vi "Excersie_3.vi"() -> ()   [LabVIEW 2013]
panel:
  in  "Slide":dbl(slide) scale=0.0..2000.0
  in  "stop":bool
  out "Waveform Chart":dbl(graph)
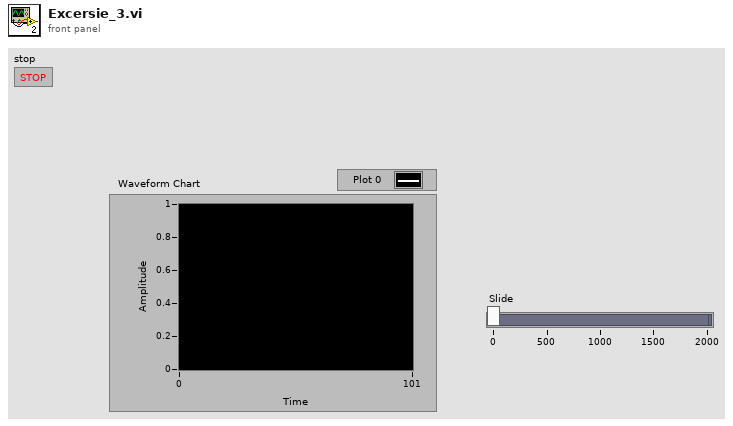
[diagram p1: front panel]
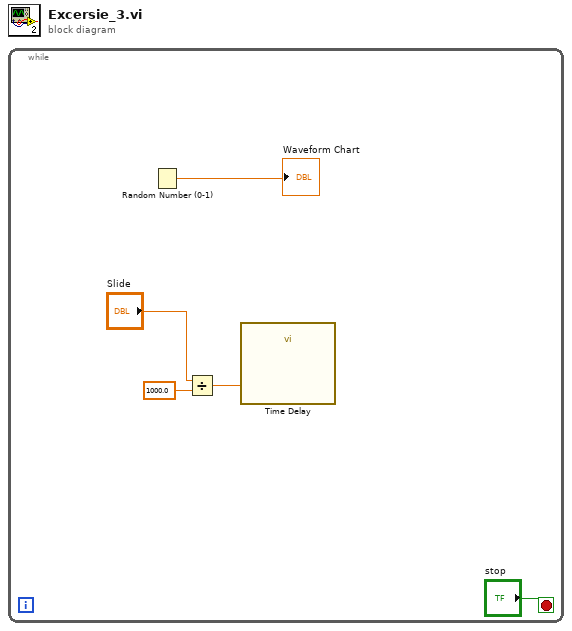
[diagram p0: block diagram]
diagram:
  n1 = while {
    stop <- "stop" stop-if-true
    n2 = Random Number (0-1)() -> (number: 0 to 1=→"Waveform Chart":dbl)
    n3 = Divide(x="Slide", y=1000.0) -> (x/y=w3:dbl)
    n4 = call "Time Delay"("Delay Time (s)"=w3) -> ()  [unwired: 10 in, 1 out]
  }
